vi "Enable SMU Output.vi"(7 "output enabled":bool=TRUE, 8 "error in (no error)":errorcluster, 10 "Channel Lists":string[](array[string]), 11 "Instrument Sessions In":refnum<k15>[](array[refnum])) -> (0 "error Out":errorcluster, 3 "Instrument Sessions Out":refnum<k15>[](array[refnum]))   [LabVIEW 2013]
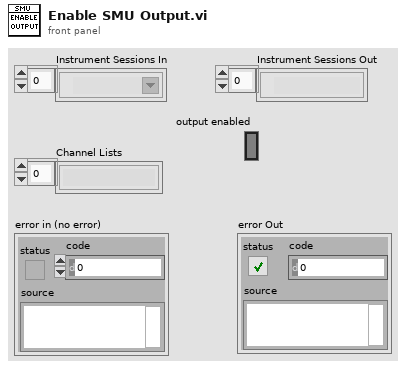
[diagram p1: front panel]
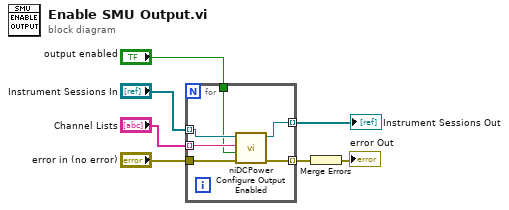
[diagram p0: block diagram]
diagram:
  n1 = for {
    tunnel: "Instrument Sessions In" -> [w13] mode=indexing
    tunnel: "Channel Lists" -> [w12] mode=indexing
    tunnel: "error in (no error)" -> [w11]
    tunnel: [w10] -> w4 mode=indexing
    tunnel: "output enabled" -> [w9]
    tunnel: [w8] -> w1 mode=indexing
    n2 = call <instrlib>:"niDCPower Configure Output Enabled.vi"("error in (no error)"=w11, "output enabled"=w9, "channel name"=w12, "instrument handle"=w13) -> ("error out"=w10:errorcluster, "instrument handle out"=w8:refnum<k15>)  [unwired: 6 in]
  }
  "Instrument Sessions Out" <- w1
  n3 = Merge Errors(w4) -> (→"error Out":errorcluster)
